vi "CDS Placement Setup.vi"   [LabVIEW 2018]
uses:
  31a7fe87-cfb1-484a-8dd2-78db81a92c1f.vi
  <vilib>/JDP Science/JSONtext/Find Item.vi
  31a7fe87-cfb1-484a-8dd2-78db81a92c1f.vi/e4a371ec-2273-4185-b51b-18f0ea440d96.vi
  <vilib>/JDP Science/JSONtext/String Subset.vi
  Wizard Config/Wizard Strings.vi
  Wizard Config/Create Default Wizard Configuration.vi
  <vilib>/JDP Science/JSONtext/Parsing/Parse Full Path or Item Name.vi
  <vilib>/JDP Science/JSONtext/Offset/Find Item Locations by Path.vi
  <vilib>/JDP Science/JSONtext/JSON text to Variant.vi
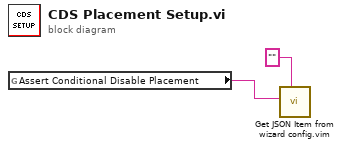
[diagram p0: block diagram]
diagram:
  n1 = global read "Wizard Strings.vi" "Assert Conditional Disable Placement"() -> (w2:string)
  n2 = call "Get JSON Item from wizard config.vim"("Data Type"="" ("$Path or Item Name"), "$Path or Item Name"=w2) -> ()  [unwired: 7 in, 3 out]
